vi "Write and Read VISA.vi"(8 "error in (no error)":errorcluster, 10 "Command to Send":string, 11 "VISA resource name in":refnum<visa-resource-name>) -> (0 "error out":errorcluster, 2 "Expected Response":string, 3 "VISA resource name out":refnum<visa-resource-name>)   [LabVIEW 2020, in "UI ACTOR.lvlib" / "UI ACTOR.lvclass"]
uses:
  UI ACTOR.lvclass
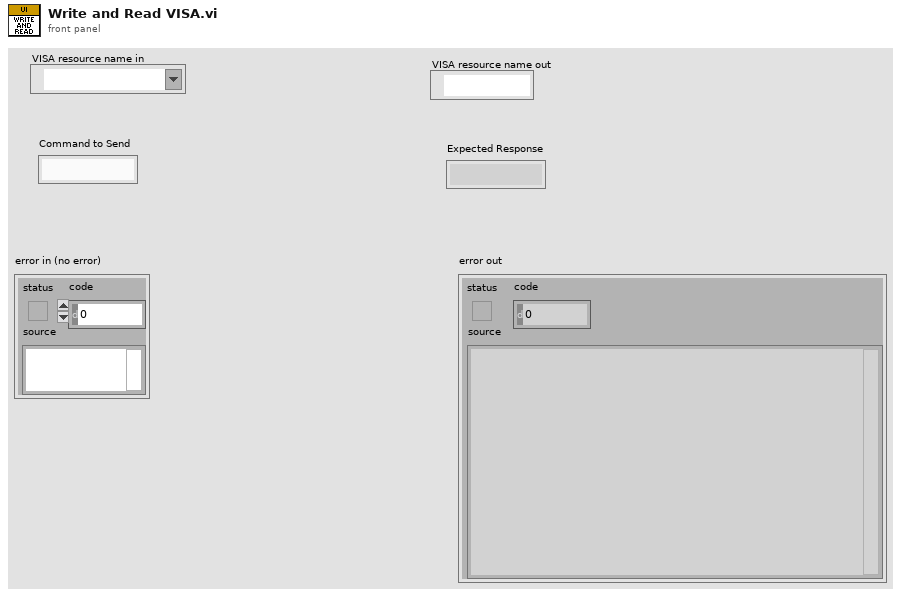
[diagram p1: front panel]
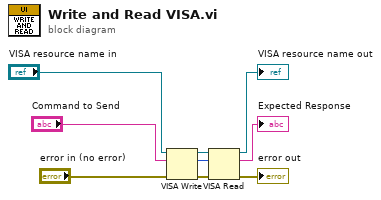
[diagram p0: block diagram]
diagram:
  n1 = VISA Write(VISA resource name="VISA resource name in", write buffer="Command to Send", error in (no error)="error in (no error)") -> (VISA resource name out=w6:refnum<visa-resource-name>, return count=w5:u32, error out=w4:errorcluster)
  n2 = VISA Read(VISA resource name=w6, byte count=w5, error in (no error)=w4) -> (VISA resource name out=→"VISA resource name out":refnum<visa-resource-name>, read buffer=→"Expected Response":string, error out=→"error out":errorcluster)  [unwired: 1 out]
